vi "Read U8.vi"(8 "error in":errorcluster, 10 "register offset":u32, 11 "session in":u32) -> (0 "error out":errorcluster, 2 "value out":u8, 3 "session out":u32)   [LabVIEW 2018, in "Scalar IO Operations.lvlib"]
uses:
  Scalar IO Operations.lvlib
  NiFpga.dll
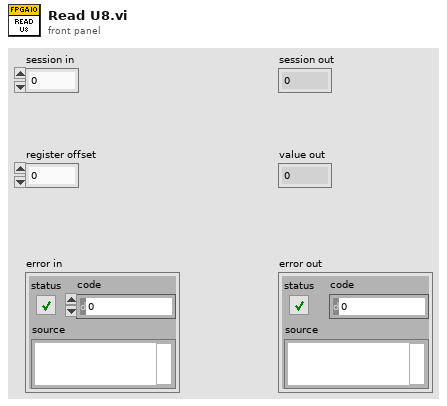
[diagram p1: front panel]
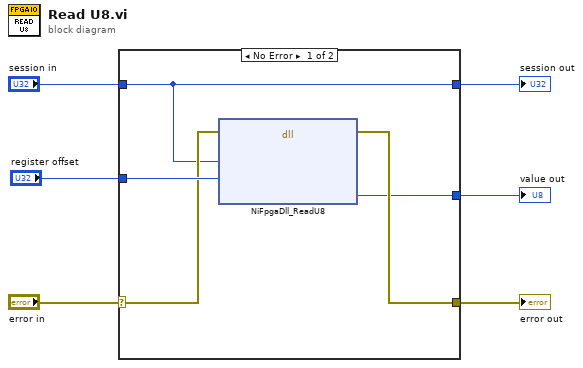
[diagram p0: block diagram]
diagram:
  n1 = case shown="No Error" "error in" {
    selector: "error in" -> [w8 w13]
    tunnel: "session in" -> [w7 w12]
    tunnel: [w11 w13] -> w5
    tunnel: [w10 _] -> w4
    tunnel: "register offset" -> [w9 _]
    tunnel: [w7 w12] -> w1
    frame No Error {
      n2 = dll-call lib="NiFpga.*" fn="NiFpgaDll_ReadU8"(error in=w8, "session"=w7, "offset"=w9) -> (error out=w11:errorcluster, "value"=w10:u8)  [unwired: 6 in, 1 out]
    }
    frame Error {
    }
  }
  "error out" <- w5
  "session out" <- w1
  "value out" <- w4
